vi "controller82.vi"(8 "Neg max speed":dbl=-1.0, 10 "reverse":bool, 11 "obs":bool) -> ()   [LabVIEW 2015]
uses:
  G_LCM.vi
  G_ALL.vi
panel:
  in  "safe_distance":dbl=1.0
  out "a_n_stop":dbl=33.53874203323456
  in  "y":dbl=100.0
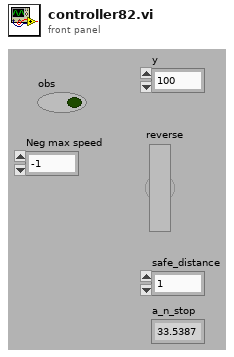
[diagram p1: front panel]
types:
  T1 = cluster{"Steer_input":dbl, "Steer_output":dbl, "VS_des":dbl, "VS_can":dbl, "heading":dbl, "auto":bool, "run":bool, "x":dbl, "y":dbl, "slam_y":dbl, "slam_x":dbl, "slam_heading":dbl}
  T2 = cluster{"hash":i64, "sys time":i64, "stopline_exist":bool, "stopline_distance":dbl}
  T3 = cluster{"hash":i64, "sys time":i64, "time":dbl, "x":dbl, "y":dbl, "h":dbl, "numSV":i32, "postype":i32, "lag":i32, "hordev":dbl, "lat":dbl, "lon":dbl, "hgt":dbl, "map_idx":i32}
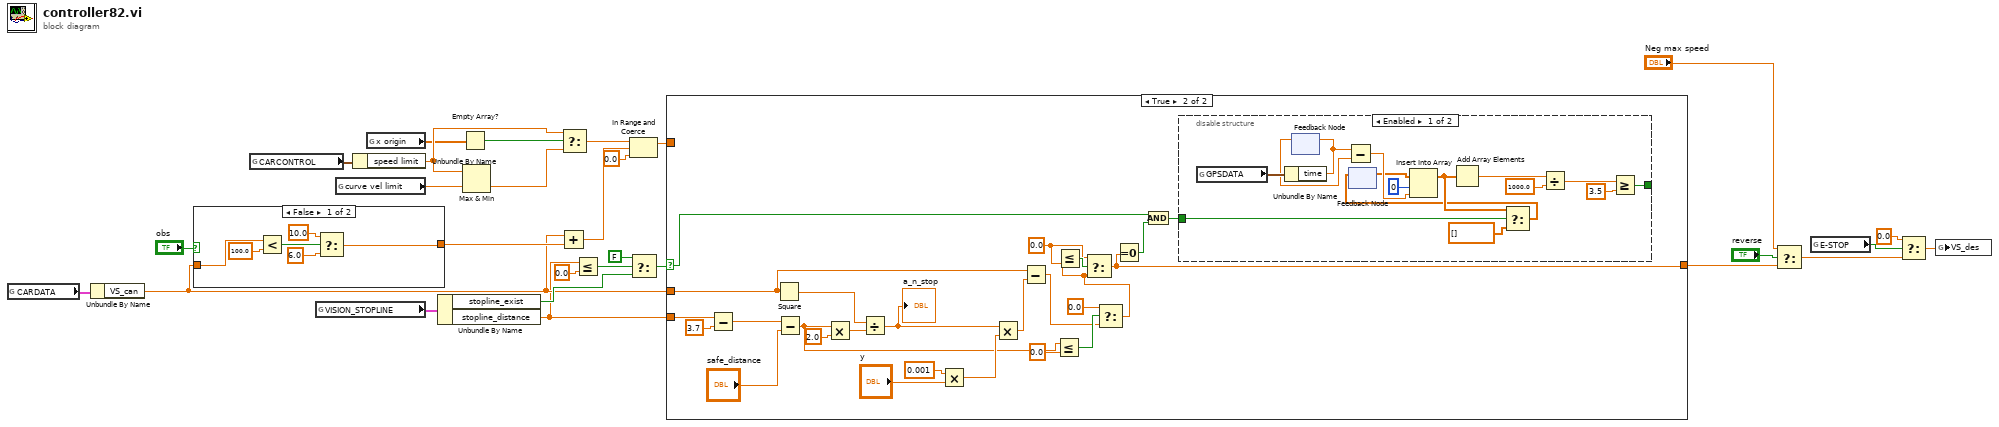
[diagram p0: block diagram]
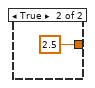
[diagram p4: hidden frame]
diagram:
  n1 = global read "G_ALL.vi" "CARDATA"() -> (w27:T1)
  n2 = Unbundle By Name(w27) -> ("VS_can"=w8:dbl)
  n3 = case shown="False" "obs" {
    tunnel: w8 -> [w34 _]
    tunnel: [w33 2.5 ("upper limit")] -> w17
    frame False {
      n4 = Less?(x=w34, y=100.0) -> (x < y?=w31:bool)
      n5 = Select(t=10.0 ("upper limit"), s=w31, f=6.0 ("upper limit")) -> (s? t:f=w33:dbl)
    }
    frame True {
    }
  }
  n6 = global read "G_ALL.vi" "CARCONTROL"() -> (w13:cluster{"speed path":dbl, "speed limit":dbl})
  n7 = global read "G_LCM.vi" "VISION_STOPLINE"() -> (w28:T2)
  n8 = global read "G_ALL.vi" "curve vel limit"() -> (w15:dbl)
  n9 = Unbundle By Name(w13) -> ("speed limit"=w20:dbl)
  n10 = global read "G_ALL.vi" "x origin"() -> (w18:dbl[])
  n11 = Unbundle By Name(w28) -> ("stopline_exist"=w25:bool, "stopline_distance"=w7:dbl)
  n12 = Empty Array?(array=w18) -> (empty?=w19:bool)
  n13 = Max & Min(x=w20, y=w15) -> (min(x,y)=w22:dbl)  [unwired: 1 out]
  n14 = Add(x=w8, y=w17) -> (x+y=w11:dbl)
  n15 = Select(t=w20, s=w19, f=w22) -> (s? t:f=w21:dbl)
  n16 = Less Or Equal?(x=w7, y=0.0) -> (x <= y?=w23:bool)
  n17 = In Range and Coerce(upper limit=w21, x=w11, lower limit=0.0) -> (coerced(x)=w5:dbl)  [unwired: 1 out]
  n18 = Select(t=FALSE, s=w23, f=w25) -> (s? t:f=w4:bool)
  n19 = case shown="True" w4 {
    selector: w4 -> [_ w45]
    tunnel: w8 -> [_ w48]
    tunnel: w7 -> [_ w49]
    tunnel: [w36 w47] -> w6
    tunnel: w5 -> [w36 _]
    frame False {
    }
    frame True {
      w50 = 0.0 ("y")
      n20 = Subtract(x=w49, y=3.7 ("x")) -> (x-y=w53:dbl)
      n21 = Square(x=w48) -> (x^2=w58:dbl)
      n22 = Subtract(x=w53, y="safe_distance") -> (x-y=w43:dbl)
      n23 = Multiply(x=w43, y=2.0) -> (x*y=w59:dbl)
      n24 = Divide(x=w58, y=w59) -> (x/y=w42:dbl)
      "a_n_stop" <- w42
      n25 = Multiply(x=0.001, y="y") -> (x*y=w56:dbl)
      n26 = Multiply(x=w42, y=w56) -> (x*y=w57:dbl)
      n27 = Subtract(x=w48, y=w57) -> (x-y=w39:dbl)
      n28 = Less Or Equal?(x=w43, y=0.0) -> (x <= y?=w40:bool)
      n29 = Select(t=0.0, s=w40, f=w39) -> (s? t:f=w37:dbl)
      n30 = Less Or Equal?(x=w37, y=w50) -> (x <= y?=w51:bool)
      n31 = Select(t=w50, s=w51, f=w37) -> (s? t:f=w47:dbl)
      n32 = Equal To 0?(x=w47) -> (x = 0?=w46:bool)
      n33 = And(x=w45, y=w46) -> (x .and. y?=w44:bool)
      n34 = disable-structure shown="Enabled" {
        disable-tunnel: [w63 _] -> _
        disable-tunnel: w44 -> [w62 _]
        frame Enabled {
          n35 = global read "G_ALL.vi" "GPSDATA"() -> (w76:T3)
          n36 = Unbundle By Name(w76) -> ("time"=w75:dbl)
          n37 = feedback #1() -> (w74:dbl)  [unwired: 1 in]
          n38 = feedback-in #1(w75) -> ()
          n39 = Subtract(x=w75, y=w74) -> (x-y=w73:dbl)
          n40 = feedback #2() -> (w67:dbl[])  [unwired: 1 in]
          n41 = Insert Into Array(array=w67, index=0, new element=w73) -> (w69:dbl[])
          n42 = Add Array Elements(numeric array=w69) -> (sum=w71:dbl)
          n43 = Select(t=w69, s=w62, f=dbl[] []) -> (s? t:f=w68:dbl[])
          n44 = feedback-in #2(w68) -> ()
          n45 = Divide(x=w71, y=1000.0) -> (x/y=w65:dbl)
          n46 = Greater Or Equal?(x=w65, y=3.5) -> (x >= y?=w63:bool)
        }
        frame Disabled {
        }
      }
    }
  }
  n47 = Select(t="Neg max speed", s="reverse", f=w6) -> (s? t:f=w16:dbl)
  n48 = global read "G_ALL.vi" "E-STOP"() -> (w12:bool)
  n49 = Select(t=0.0, s=w12, f=w16) -> (s? t:f=w14:dbl)
  n50 = global write "G_ALL.vi" "VS_des"(w14) -> ()
